vi "PicoScope4000aExampleAdvancedTrigger.vi"() -> ()   [LabVIEW 2010]
uses:
  shared/PicoBuffers.ctl
  PicoScope4000aLib/PicoScope4000aAnalogChannelSettings.ctl
  shared/Buffer and Transfer Settings.ctl
  shared/Acquisition Settings.ctl
panel:
  out "Unit Info":T1={"Driver Version"="2.1.116.3546", "USB Version"="3.0", "Hardware"="1", "Variant"="4824A", "Batch and Serial"="ZZ990/003", "Cal Date"="19Dec13", "Kernel Version"="1.0", "Digital HW Version"="1", "Analogue HW Version"="1", "Firmware 1"="1.8.2.0", "Firmware 2"="1.0.12.0", "Num. channels"=8}
  in  "Pulse Width Qualifier Conditions":T2 {"Channel H" items=["Don't Care", "True", "False"]; "Channel G" items=["Don't Care", "True", "False"]; "Channel F" items=["Don't Care", "True", "False"]; "Channel E" items=["Don't Care", "True", "False"]; "Aux" items=["Don't Care", "True", "False"]; "Ext" items=["Don't Care", "True", "False"]; "Channel D" items=["Don't Care", "True", "False"]; "Channel C" items=["Don't Care", "True", "False"]; "Channel B" items=["Don't Care", "True", "False"]; "Channel A" items=["Don't Care", "True", "False"]; "Condition Logic" items=["AND", "OR", "XOR"]}
  in  "Channel B Settings":T3={"Enabled"=FALSE, "Coupling"=1, "Range"=6, "Analogue Offset"=0.0, "Bandwidth Limit"=0} {"Bandwidth Limit" items=["Full", "20kHz", "100kHz", "1MHz"]; "Range" items=["10 mV", "20 mV", "50 mV", "100 mV", "200 mV", "500 mV", "1 V", "2 V", "5 V", "10 V", "20 V", "50 V ", "100 V"]; "Coupling" items=["AC", "DC"]}
  in  "Pulse Width Qualifier Settings":T4={"Direction"=2, "Lower Limit"=0, "Upper Limit"=0, "Pulse Width Type"=0} {"Pulse Width Type" items=["None", "Less Than", "Greater Than", "In Range", "Out of Range"]; "Direction" items=["Rising"=2, "Falling"=3, "Rising Lower"=7, "Above"=0, "Below"=1, "Rising or Falling"=4, "Falling Lower"=8, "Below Lower"=6, "Above Lower"=5]}
  in  "Auto Trigger (ms)":i32=1000
  in  "Channel Trigger Properties":T5={"Channel A Trigger Properties"={"thresholdUpper"=0, "thresholdUpperHysteresis"=0, "thresholdLower"=0, "thresholdLowerHysteresis"=0, "Threshold Mode"=0, "Direction"=2, "Available"=TRUE}, "Channel B Trigger Properties"={"thresholdUpper"=0, "thresholdUpperHysteresis"=0, "thresholdLower"=0, "thresholdLowerHysteresis"=0, "Threshold Mode"=0, "Direction"=2, "Available"=FALSE}, "Channel C Trigger Properties"={"thresholdUpper"=0, "thresholdUpperHysteresis"=0, "thresholdLower"=0, "thresholdLowerHysteresis"=0, "Threshold Mode"=0, "Direction"=2, "Available"=FALSE}, "Channel D Trigger Properties"={"thresholdUpper"=0, "thresholdUpperHysteresis"=0, "thresholdLower"=0, "thresholdLowerHysteresis"=0, "Threshold Mode"=0, "Direction"=2, "Available"=FALSE}, "Channel E Trigger Properties"={"thresholdUpper"=0, "thresholdUpperHysteresis"=0, "thresholdLower"=0, "thresholdLowerHysteresis"=0, "Threshold Mode"=0, "Direction"=2, "Available"=FALSE}, "Channel F Trigger Properties"={"thresholdUpper"=0, "thresholdUpperHysteresis"=0, "thresholdLower"=0, "thresholdLowerHysteresis"=0, "Threshold Mode"=0, "Direction"=2, "Available"=FALSE}, "Channel G Trigger Properties"={"thresholdUpper"=0, "thresholdUpperHysteresis"=0, "thresholdLower"=0, "thresholdLowerHysteresis"=0, "Threshold Mode"=0, "Direction"=2, "Available"=FALSE}, "Channel H Trigger Properties"={"thresholdUpper"=0, "thresholdUpperHysteresis"=0, "thresholdLower"=0, "thresholdLowerHysteresis"=0, "Threshold Mode"=0, "Direction"=2, "Available"=FALSE}} {"Channel H Trigger Properties"."Direction" items=["Above / Inside", "Below / Outside", "Rising / Enter", "Falling / Exit", "Rising or Falling / Enter or Exit", "Above Lower", "Below Lower", "Rising Lower", "Falling Lower", "Positive Runt", "Negative Runt"]; "Channel H Trigger Properties"."Threshold Mode" items=["Level", "Window"]; "Channel G Trigger Properties"."Direction" items=["Above / Inside", "Below / Outside", "Rising / Enter", "Falling / Exit", "Rising or Falling / Enter or Exit", "Above Lower", "Below Lower", "Rising Lower", "Falling Lower", "Positive Runt", "Negative Runt"]; "Channel G Trigger Properties"."Threshold Mode" items=["Level", "Window"]; "Channel F Trigger Properties"."Direction" items=["Above / Inside", "Below / Outside", "Rising / Enter", "Falling / Exit", "Rising or Falling / Enter or Exit", "Above Lower", "Below Lower", "Rising Lower", "Falling Lower", "Positive Runt", "Negative Runt"]; "Channel F Trigger Properties"."Threshold Mode" items=["Level", "Window"]; "Channel E Trigger Properties"."Direction" items=["Above / Inside", "Below / Outside", "Rising / Enter", "Falling / Exit", "Rising or Falling / Enter or Exit", "Above Lower", "Below Lower", "Rising Lower", "Falling Lower", "Positive Runt", "Negative Runt"]; "Channel E Trigger Properties"."Threshold Mode" items=["Level", "Window"]; "Channel D Trigger Properties"."Direction" items=["Above / Inside", "Below / Outside", "Rising / Enter", "Falling / Exit", "Rising or Falling / Enter or Exit", "Above Lower", "Below Lower", "Rising Lower", "Falling Lower", "Positive Runt", "Negative Runt"]; "Channel D Trigger Properties"."Threshold Mode" items=["Level", "Window"]; "Channel C Trigger Properties"."Direction" items=["Above / Inside", "Below / Outside", "Rising / Enter", "Falling / Exit", "Rising or Falling / Enter or Exit", "Above Lower", "Below Lower", "Rising Lower", "Falling Lower", "Positive Runt", "Negative Runt"]; "Channel C Trigger Properties"."Threshold Mode" items=["Level", "Window"]; "Channel B Trigger Properties"."Direction" items=["Above / Inside", "Below / Outside", "Rising / Enter", "Falling / Exit", "Rising or Falling / Enter or Exit", "Above Lower", "Below Lower", "Rising Lower", "Falling Lower", "Positive Runt", "Negative Runt"]; "Channel B Trigger Properties"."Threshold Mode" items=["Level", "Window"]; "Channel A Trigger Properties"."Direction" items=["Above / Inside", "Below / Outside", "Rising / Enter", "Falling / Exit", "Rising or Falling / Enter or Exit", "Above Lower", "Below Lower", "Rising Lower", "Falling Lower", "Positive Runt", "Negative Runt"]; "Channel A Trigger Properties"."Threshold Mode" items=["Level", "Window"]}
  in  "Trigger Conditions":T6={"Channel A"=1, "Channel B"=0, "Channel C"=0, "Channel D"=0, "Channel E"=0, "Channel F"=0, "Channel G"=0, "Channel H"=0, "Ext"=0, "Aux"=0, "PWQ"=0, "Condition Logic"=0} {"Channel H" items=["Don't Care", "True", "False"]; "Channel G" items=["Don't Care", "True", "False"]; "Channel F" items=["Don't Care", "True", "False"]; "Channel E" items=["Don't Care", "True", "False"]; "PWQ" items=["Don't Care", "True", "False"]; "Aux" items=["Don't Care", "True", "False"]; "Ext" items=["Don't Care", "True", "False"]; "Channel D" items=["Don't Care", "True", "False"]; "Channel C" items=["Don't Care", "True", "False"]; "Channel B" items=["Don't Care", "True", "False"]; "Channel A" items=["Don't Care", "True", "False"]; "Condition Logic" items=["AND", "OR", "XOR"]}
  in  "Resolution":u32(ring)=1 items=["8-bit", "12-bit", "14-bit"]
  out "overflow":i16 format="%08b"
  in  "Apply Settings":bool
  in  "Channel A Settings":T3={"Enabled"=TRUE, "Coupling"=1, "Range"=6, "Analogue Offset"=0.0, "Bandwidth Limit"=0} {"Bandwidth Limit" items=["Full", "20kHz", "100kHz", "1MHz"]; "Range" items=["10 mV", "20 mV", "50 mV", "100 mV", "200 mV", "500 mV", "1 V", "2 V", "5 V", "10 V", "20 V", "50 V ", "100 V"]; "Coupling" items=["AC", "DC"]}
  out "USB 3.0 device on non-USB 3.0 Port":bool
  out "USB Powered":bool=TRUE
  out "error out":errorcluster
  in  "Data file":path=path "PicoScope4000aExampleAdvancetrigger ChA Data"
  in  "Buffer and Transfer Settings":T7={"startIndex"=0, "Samples"=2000000, "Down Sample Ratio"=1, "Down-Sample Mode"=0} {"Down-Sample Mode" items=["RAW none"=2147483648, "None"=0, "Aggregate"=1, "Decimate"=2, "Average"=4]; "Down Sample Ratio" step=1; "Samples" format="%_6p"}
  in  "Acquisition Settings":T8={"preTriggerSamples"=1000000, "postTriggerSamples"=1000000, "timebase"=5} {"postTriggerSamples" format="%_6p"; "preTriggerSamples" format="%_6p"}
  out "Properties Panel":T9={"Sample Frequency"=13333333.333333334, "Sample Rate"=7.5e-08, "Max Samples Available"=268435264, "Number of Samples"=0, "Total Capture Time (sec) "=0.0, "Max Total Capture Time Available (sec)"=20.132644799999998} {"Max Total Capture Time Available (sec)" format="%.3p"; "Sample Frequency" format="%.6p"; "Sample Rate" format="%.3p"; "Max Samples Available" format="%_6p"; "Total Capture Time (sec)" format="%.3p"}
  in  "stop":bool
  out "Analog Channels":cluster{i32, dbl, "Data":dbl[]}[](graph)
  in  "Serial Number":string
  in  "Use Serial Number":bool
  in  "error in (no error)":errorcluster
  # "Bit 0 = ChA"
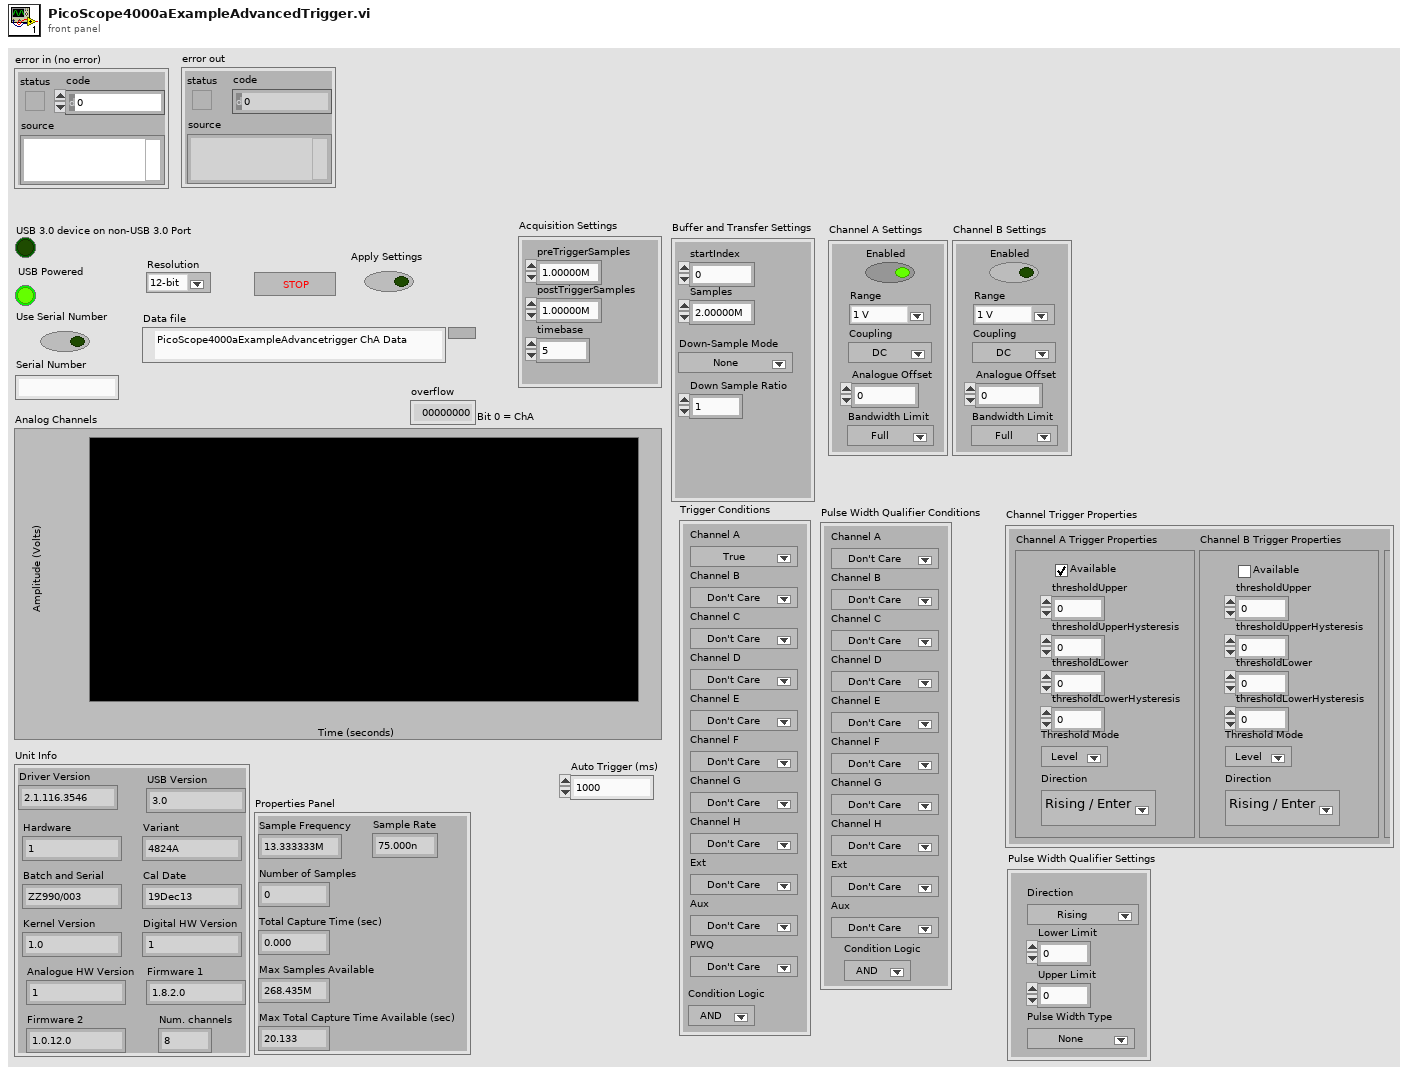
[diagram p1: front panel]
types:
  T1 = cluster{"Driver Version":string, "USB Version":string, "Hardware":string, "Variant":string, "Batch and Serial":string, "Cal Date":string, "Kernel Version":string, "Digital HW Version":string, "Analogue HW Version":string, "Firmware 1":string, "Firmware 2":string, "Num. channels":i16}
  T2 = cluster{"Channel A":u16, "Channel B":u16, "Channel C":u16, "Channel D":u16, "Channel E":u16, "Channel F":u16, "Channel G":u16, "Channel H":u16, "Ext":u16, "Aux":u16, "Condition Logic":u16}
  T3 = typedef "PicoScope4000aAnalogChannelSettings.ctl" = cluster{"Enabled":bool, "Coupling":i16, "Range":u32, "Analogue Offset":sgl, "Bandwidth Limit":u32}
  T4 = cluster{"Direction":u32, "Lower Limit":u32, "Upper Limit":u32, "Pulse Width Type":u32}
  T5 = cluster{"Channel A Trigger Properties":cluster{"thresholdUpper":i16, "thresholdUpperHysteresis":u16, "thresholdLower":i16, "thresholdLowerHysteresis":u16, "Threshold Mode":i32, "Direction":i32, "Available":bool}, "Channel B Trigger Properties":cluster{"thresholdUpper":i16, "thresholdUpperHysteresis":u16, "thresholdLower":i16, "thresholdLowerHysteresis":u16, "Threshold Mode":i32, "Direction":i32, "Available":bool}, "Channel C Trigger Properties":cluster{"thresholdUpper":i16, "thresholdUpperHysteresis":u16, "thresholdLower":i16, "thresholdLowerHysteresis":u16, "Threshold Mode":i32, "Direction":i32, "Available":bool}, "Channel D Trigger Properties":cluster{"thresholdUpper":i16, "thresholdUpperHysteresis":u16, "thresholdLower":i16, "thresholdLowerHysteresis":u16, "Threshold Mode":i32, "Direction":i32, "Available":bool}, "Channel E Trigger Properties":cluster{"thresholdUpper":i16, "thresholdUpperHysteresis":u16, "thresholdLower":i16, "thresholdLowerHysteresis":u16, "Threshold Mode":i32, "Direction":i32, "Available":bool}, "Channel F Trigger Properties":cluster{"thresholdUpper":i16, "thresholdUpperHysteresis":u16, "thresholdLower":i16, "thresholdLowerHysteresis":u16, "Threshold Mode":i32, "Direction":i32, "Available":bool}, "Channel G Trigger Properties":cluster{"thresholdUpper":i16, "thresholdUpperHysteresis":u16, "thresholdLower":i16, "thresholdLowerHysteresis":u16, "Threshold Mode":i32, "Direction":i32, "Available":bool}, "Channel H Trigger Properties":cluster{"thresholdUpper":i16, "thresholdUpperHysteresis":u16, "thresholdLower":i16, "thresholdLowerHysteresis":u16, "Threshold Mode":i32, "Direction":i32, "Available":bool}}
  T6 = cluster{"Channel A":u16, "Channel B":u16, "Channel C":u16, "Channel D":u16, "Channel E":u16, "Channel F":u16, "Channel G":u16, "Channel H":u16, "Ext":u16, "Aux":u16, "PWQ":u16, "Condition Logic":u16}
  T7 = typedef "Buffer and Transfer Settings.ctl" = cluster{"startIndex":u64, "Samples":u64, "Down Sample Ratio":u64, "Down-Sample Mode":u32}
  T8 = typedef "Acquisition Settings.ctl" = cluster{"preTriggerSamples":u64, "postTriggerSamples":u64, "timebase":u32}
  T9 = cluster{"Sample Frequency":dbl, "Sample Rate":dbl, "Max Samples Available":u64, "Number of Samples":u64, "Total Capture Time (sec) ":dbl, "Max Total Capture Time Available (sec)":dbl}
  T10 = enum16{"open", "open or create", "create or replace", "create", "open (read-only)"}
  T11 = typedef "PicoBuffers.ctl" = cluster{"Max Buffer Pointers":u64[][][], "Min Buffer Pointers":u64[][][], "StreamingDataInfo":cluster{"Channel":u32, "Down-Sample Mode":u32, "PICO_DATA_TYPE":enum32{"PICO_INT8_T", "PICO_INT16_T", "PICO_INT32_T", "PICO_UINT32_T", "PICO_INT64_T", ""}, "Samples":i32, "bufferIndex":u64, "startIndex":i32, "overflow":i16}[][]}
  T12 = cluster{"Channel A Buffer":i16[], "Channel B Buffer":i16[], "Channel C Buffer":i16[], "Channel D Buffer":i16[], "Channel E Buffer":i16[], "Channel F Buffer":i16[], "Channel G Buffer":i16[], "Channel H Buffer":i16[], "Port 0 Buffer":i16[], "Port 1 Buffer":i16[]}[]
  T13 = cluster{"Channel A Buffer":i16[], "Channel B Buffer":i16[], "Channel C Buffer":i16[], "Channel D Buffer":i16[], "Channel E Buffer":i16[], "Channel F Buffer":i16[], "Channel G Buffer":i16[], "Channel H Buffer":i16[], "Port 0 Buffer":i16[], "Port 1 Buffer":i16[]}
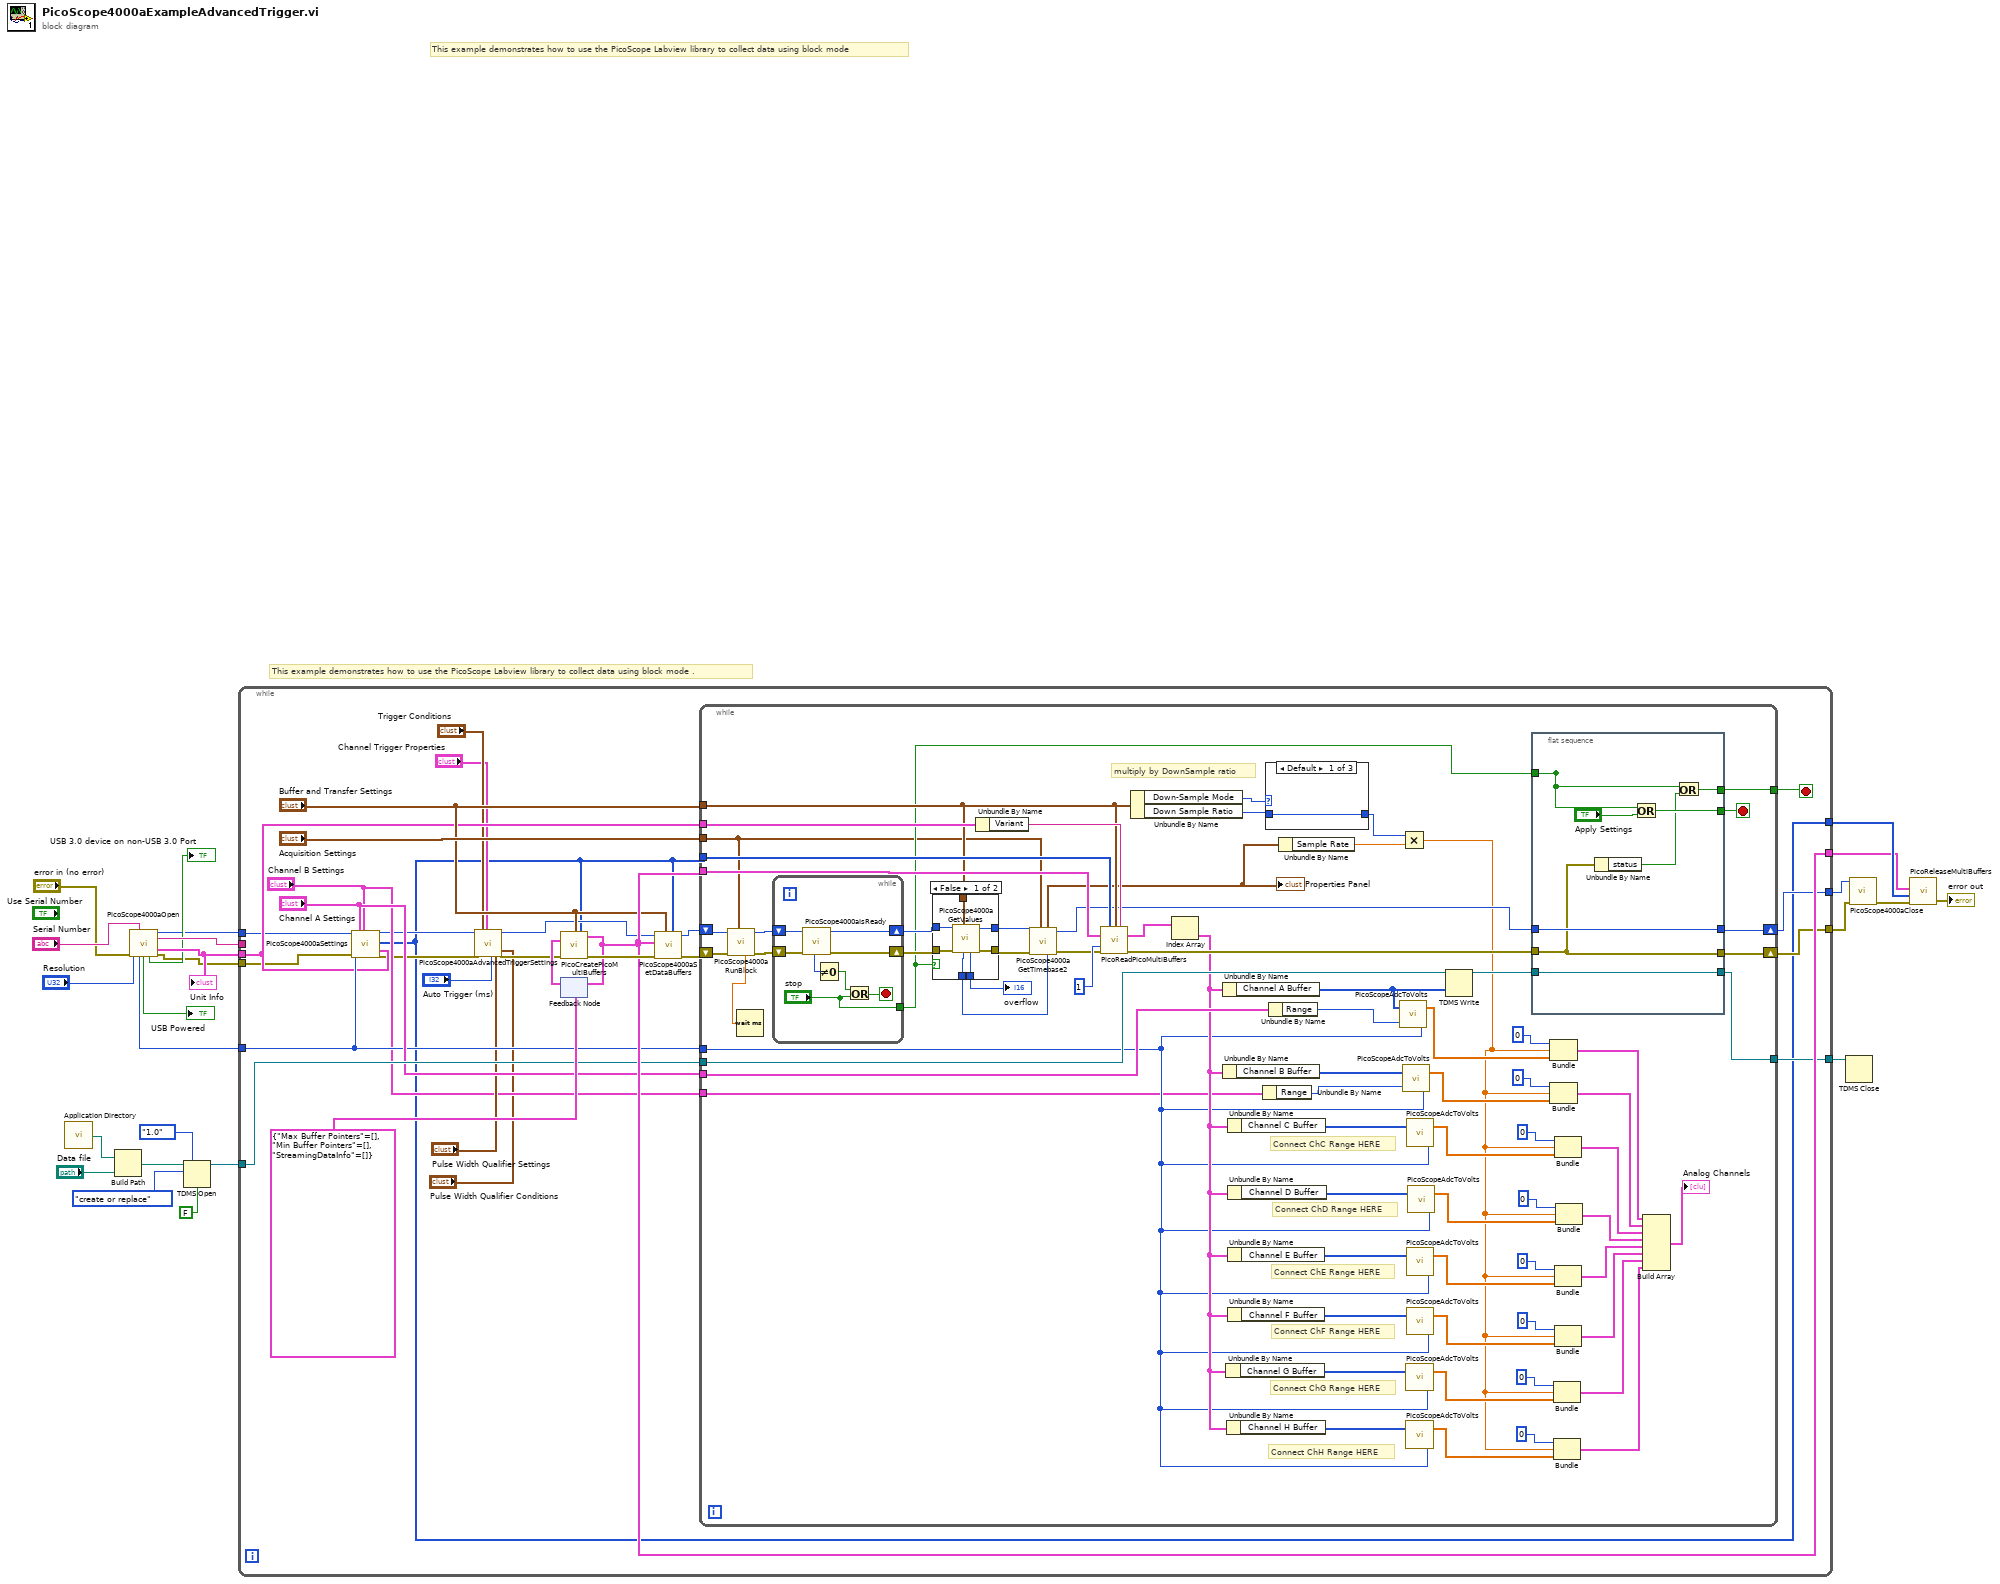
[diagram p0: block diagram]
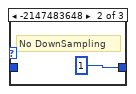
[diagram p3: hidden frame]
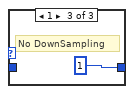
[diagram p4: hidden frame]
diagram:
  # "This example demonstrates how to use the PicoScope Labview library to collect data using block mode ."
  # "This example demonstrates how to use the PicoScope Labview library to collect data using block mode"
  n1 = call <vilib>:"Application Directory.vi"() -> ("Application Directory"=w17:path)
  n2 = Build Path(base path=w17, name or relative path="Data file") -> (appended path=w18:path)
  n3 = call "PicoScope4000aOpen.vi"("Serial Number"="Serial Number", "Resolution"="Resolution", "error in (no error)"="error in (no error)") -> ("handle"=w7:i16, "Pico 4000a Units"=w10:string, "Unit Info"=w11:T1, "Max ADC value"=w13:i16, "USB powered"=→"USB Powered":bool, "USB 3.0 on non-USB 3.0 port"=→"USB 3.0 device on non-USB 3.0 Port":bool, "error out"=w1:errorcluster)  [unwired: 5 in, 1 out]
  "Unit Info" <- w11
  n4 = TDMS Open(6:FALSE ("disable buffering? (T)"), 7:enum16{"1.0", "2.0"}."1.0" ("file format version (2.0)"), 10:T10."create or replace" ("operation (0:open)"), 11:w18) -> (3:w15:refnum<k34>)  [unwired: 2 in, 1 out]
  n5 = while {
    tunnel: w10 -> [_]
    tunnel: w13 -> [w46]
    tunnel: [w25] -> w24
    tunnel: [w50] -> w23
    tunnel: [w44] -> w16
    tunnel: w15 -> [w49]
    tunnel: w7 -> [w29]
    tunnel: [w45] -> w4
    tunnel: [w42] -> w12
    tunnel: w11 -> [w38]
    tunnel: w1 -> [w28]
    stop <- w43 stop-if-true
    n6 = call "PicoScope4000aSettings.vi"("handle in"=w29, "Max ADC value"=w46, "error in"=w28, "Channel A Settings"="Channel A Settings", "Channel B Settings"="Channel B Settings", "Unit Info"=w38) -> ("handle out"=w27:i16, "Enabled array"=w25:i16[], "error out"=w26:errorcluster)  [unwired: 11 in]
    n7 = call "PicoScope4000aAdvancedTriggerSettings.vi"("handle in"=w27, "error in"=w26, "Trigger Conditions"="Trigger Conditions", "Channel Trigger Properties"="Channel Trigger Properties", "Auto Trigger (ms)"="Auto Trigger (ms)", "Pulse Width Qualifier Conditions"="Pulse Width Qualifier Conditions", "Pulse Width Qualifier Settings"="Pulse Width Qualifier Settings") -> ("handle out"=w36:i16, "error out"=w37:errorcluster)  [unwired: 11 in]
    n8 = feedback #1(T11 {"Max Buffer Pointers"=[], "Min Buffer Pointers"=[], "StreamingDataInfo"=[]} ("Data Pointers")) -> (w52:T11)
    n9 = call "PicoCreatePicoMultiBuffers.vi"("Buffer and Transfer Settings"="Buffer and Transfer Settings", "enabled array"=w25, "Data Pointers In"=w52, "error in (no error)"=w37) -> ("Data Pointers"=w50:T11, "error out"=w51:errorcluster)  [unwired: 10 in]
    n10 = feedback-in #1(w50) -> ()
    n11 = call "PicoScope4000aSetDataBuffers.vi"("enabled array"=w25, "Buffer and Transfer Settings"="Buffer and Transfer Settings", "error in (no error)"=w51, "Data Pointers In"=w50, "handle in"=w36) -> ("error out"=w41:errorcluster, "handle out"=w40:i16)  [unwired: 5 in]
    n12 = while {
      tunnel: w50 -> [w128]
      tunnel: "Buffer and Transfer Settings" -> [w85]
      tunnel: w25 -> [w120]
      tunnel: "Channel A Settings" -> [w119]
      tunnel: "Acquisition Settings" -> [w76]
      tunnel: w46 -> [w62]
      tunnel: w38 -> [w116]
      tunnel: [w92] -> w43
      shift-right: [w96] -> w45
      shift-left: w41 -> [w86]
      shift-right: [w90] -> w42
      shift-left: w40 -> [w87]
      tunnel: w49 -> [w127]
      tunnel: [w94] -> w44
      tunnel: "Channel B Settings" -> [w54]
      stop <- w91 stop-if-true
      # "Connect ChH Range HERE"
      # "Connect ChG Range HERE"
      # "Connect ChF Range HERE"
      # "Connect ChE Range HERE"
      # "Connect ChD Range HERE"
      # "Connect ChC Range HERE"
      # "multiply by DownSample ratio"
      n13 = call "PicoScope4000aRunBlock.vi"("Acquisition Settings"=w76, "error in (no error)"=w86, "handle in"=w87) -> ("error out"=w122:errorcluster, "handle out"=w121:i16, "timeIndisposedMs"=w56:dbl)  [unwired: 5 in, 1 out]
      n14 = Wait (ms)(milliseconds to wait=w56) -> ()  [unwired: 1 out]
      n15 = while {
        shift-right: [w152] -> w88
        shift-left: w122 -> [w153]
        shift-right: [w151] -> w89
        shift-left: w121 -> [w150]
        tunnel: ["stop"] -> w84
        stop <- w147 stop-if-true
        n16 = call "PicoScope4000aIsReady.vi"("error in (no error)"=w153, "handle in"=w150) -> ("error out"=w152:errorcluster, "handle out"=w151:i16, "ready"=w149:i16)  [unwired: 7 in]
        n17 = Not Equal To 0?(x=w149) -> (x != 0?=w148:bool)
        n18 = Or(x=w148, y="stop") -> (x .or. y?=w147:bool)
      }
      n19 = case shown="False" w84 {
        tunnel: w88 -> [w135 w136]
        tunnel: w89 -> [w134 w137]
        tunnel: [w133 w137] -> w78
        tunnel: [w132 w136] -> w79
        tunnel: w85 -> [w131 _]
        tunnel: [w130 _] -> w83
        tunnel: [w129 _] -> w82
        frame False {
          n20 = call "PicoScope4000aGetValues.vi"("Buffer and Transfer Settings"=w131, "error in (no error)"=w135, "handle in"=w134) -> ("error out"=w132:errorcluster, "handle out"=w133:i16, "overflow"=w130:i16, "noOfSamples"=w129:u64)  [unwired: 5 in]
        }
        frame True {
        }
      }
      "overflow" <- w83
      n21 = Unbundle By Name(w116) -> ("Variant"=w117:string)
      n22 = call "PicoScope4000aGetTimebase2.vi"("Number of Samples"=w82, "Acquisition Settings"=w76, "error in (no error)"=w79, "handle in"=w78) -> ("error out"=w80:errorcluster, "handle out"=w77:i16, "Properties Panel"=w81:T9)  [unwired: 5 in]
      "Properties Panel" <- w81
      n23 = call "PicoReadPicoMultiBuffers.vi"("enabled array"=w120, "Buffer and Transfer Settings"=w85, "Variant"=w117, "Data Pointers"=w128, "No of Buffers"=1, "error in (no error)"=w80) -> ("MultiBuffers (Max or non-aggregated)"=w126:T12, "error out"=w93:errorcluster)  [unwired: 7 in, 1 out]
      n24 = Unbundle By Name(w85) -> ("Down-Sample Mode"=w124:u32, "Down Sample Ratio"=w125:u64)
      n25 = Index Array(array=w126) -> (element=w63:T13)  [unwired: 1 in]
      n26 = Unbundle By Name(w63) -> ("Channel A Buffer"=w105:i16[])
      n27 = Unbundle By Name(w63) -> ("Channel B Buffer"=w111:i16[])
      n28 = Unbundle By Name(w63) -> ("Channel G Buffer"=w68:i16[])
      n29 = Unbundle By Name(w63) -> ("Channel H Buffer"=w65:i16[])
      n30 = Unbundle By Name(w63) -> ("Channel C Buffer"=w103:i16[])
      n31 = Unbundle By Name(w63) -> ("Channel D Buffer"=w99:i16[])
      n32 = Unbundle By Name(w63) -> ("Channel E Buffer"=w74:i16[])
      n33 = Unbundle By Name(w63) -> ("Channel F Buffer"=w71:i16[])
      n34 = Unbundle By Name(w54) -> ("Range"=w55:u32)
      n35 = case shown="Default" w124 {
        tunnel: [w154 u64 1 ("Down Sample Ratio") u64 1 ("Down Sample Ratio")] -> w123
        tunnel: w125 -> [w154 _ _]
        frame Default {
        }
        frame -2147483648 {
          # "No DownSampling"
        }
        frame 1 {
          # "No DownSampling"
        }
      }
      n36 = Unbundle By Name(w119) -> ("Range"=w113:u32)
      n37 = Unbundle By Name(w81) -> ("Sample Rate"=w118:dbl)
      n38 = call "PicoScopeAdcToVolts.vi"("Max_adc"=w62, "Range Index"=w113, "Data"=w105) -> ("Data"=w106:dbl[])
      n39 = Multiply(x=w123, y=w118) -> (x*y=w60:dbl)
      n40 = call "PicoScopeAdcToVolts.vi"("Max_adc"=w62, "Range Index"=w55, "Data"=w111) -> ("Data"=w110:dbl[])
      n41 = call "PicoScopeAdcToVolts.vi"("Max_adc"=w62, "Data"=w68) -> ("Data"=w67:dbl[])  [unwired: 1 in]
      n42 = call "PicoScopeAdcToVolts.vi"("Max_adc"=w62, "Data"=w65) -> ("Data"=w64:dbl[])  [unwired: 1 in]
      n43 = call "PicoScopeAdcToVolts.vi"("Max_adc"=w62, "Data"=w103) -> ("Data"=w102:dbl[])  [unwired: 1 in]
      n44 = call "PicoScopeAdcToVolts.vi"("Max_adc"=w62, "Data"=w74) -> ("Data"=w73:dbl[])  [unwired: 1 in]
      n45 = call "PicoScopeAdcToVolts.vi"("Max_adc"=w62, "Data"=w71) -> ("Data"=w70:dbl[])  [unwired: 1 in]
      n46 = call "PicoScopeAdcToVolts.vi"("Max_adc"=w62, "Data"=w99) -> ("Data"=w98:dbl[])  [unwired: 1 in]
      n47 = TDMS Write(0:w127, 9:w105) -> (4:w95:refnum<k34>)  [unwired: 4 in, 3 out]
      n48 = flat-sequence {
        tunnel: [w145] -> w91
        tunnel: [w138] -> _
        tunnel: [w142] -> w92
        tunnel: w77 -> [w141]
        tunnel: [w141] -> w90
        tunnel: w93 -> [w140]
        tunnel: [w140] -> w96
        tunnel: [w139] -> w94
        tunnel: w95 -> [w139]
        tunnel: w84 -> [w138]
        frame #0 {
          n49 = Unbundle By Name(w140) -> ("status"=w143:bool)
          n50 = Or(x=w138, y="Apply Settings") -> (x .or. y?=w145:bool)
          n51 = Or(x=w138, y=w143) -> (x .or. y?=w142:bool)
        }
      }
      n52 = Bundle(0, w60, "Data"=w106) -> (w109:cluster{i32, dbl, "Data":dbl[]})  [unwired: 1 in]
      n53 = Bundle(0, w60, "Data"=w110) -> (w108:cluster{i32, dbl, "Data":dbl[]})  [unwired: 1 in]
      n54 = Bundle(0, w60, "Data"=w67) -> (w58:cluster{i32, dbl, "Data":dbl[]})  [unwired: 1 in]
      n55 = Bundle(0, w60, "Data"=w64) -> (w57:cluster{i32, dbl, "Data":dbl[]})  [unwired: 1 in]
      n56 = Bundle(0, w60, "Data"=w102) -> (w101:cluster{i32, dbl, "Data":dbl[]})  [unwired: 1 in]
      n57 = Bundle(0, w60, "Data"=w73) -> (w61:cluster{i32, dbl, "Data":dbl[]})  [unwired: 1 in]
      n58 = Bundle(0, w60, "Data"=w70) -> (w59:cluster{i32, dbl, "Data":dbl[]})  [unwired: 1 in]
      n59 = Bundle(0, w60, "Data"=w98) -> (w97:cluster{i32, dbl, "Data":dbl[]})  [unwired: 1 in]
      n60 = Build Array(w109, w108, w101, w97, w61, w59, w58, w57) -> (→"Analog Channels":cluster{i32, dbl, "Data":dbl[]}[])
    }
  }
  n61 = TDMS Close(11:w16) -> ()  [unwired: 1 in, 2 out]
  n62 = call "PicoScope4000aClose.vi"("error in (no error)"=w4, "handle in"=w12) -> ("error out"=w3:errorcluster)  [unwired: 7 in, 1 out]
  n63 = call "PicoReleaseMultiBuffers.vi"("error in (no error)"=w3, "Enabled array"=w24, "Data Pointers"=w23) -> ("error out"=→"error out":errorcluster)  [unwired: 7 in, 1 out]
